vi "Image Dispose.vi"(5 "Archive?":bool, 7 "Dispose?":bool, 8 "error in":errorcluster, 11 "Gluing Procedure in":refnum<class "Gluing Procedure.lvclass">) -> (0 "error out":errorcluster, 3 "Gluing Procedure out":refnum<class "Gluing Procedure.lvclass">)   [LabVIEW 2017, in "Gluing Procedure.lvclass"]
uses:
  Gluing Procedure.lvclass
  Shared Components/Gantry Class/Gantry Class.lvclass
  Shared Components/Config Manager Class/Config Manager Class.lvclass
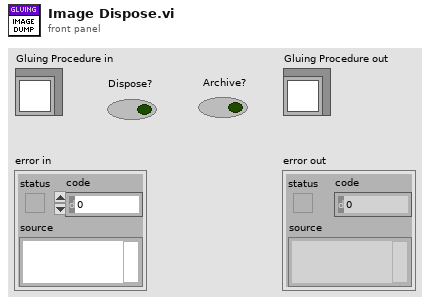
[diagram p1: front panel]
types:
  T1 = typedef "Part Fiducials.ctl" = cluster{"Fiducials":T2[], "Chuck":i32, "Slot":i32}
  T2 = typedef "Fiducial Image.ctl" = cluster{"Fiducial Image":T3, "Selected Fiducial":T5, "fiducial name":string}
  T3 = typedef "Physical Image.ctl" = cluster{"Image Position":refnum<class "Vec3d Class.lvclass">, "Image Reference":T4, "Field of View":cluster{"x(mm)":dbl, "y(mm)":dbl}}
  T4 = typedef "IMAQ Image.ctl" = refnum<image>
  T5 = typedef "Fiducial with Source.ctl" = cluster{"Fiducial Image Coordinate":refnum<class "Vec3d Class.lvclass">, "Fiducial Source":enum16{"Pattern Recognition", "User", "Error", "Default"}}
  T6 = cluster{"HDI Fiducials":T1, "Stamp Fiducials":T1, "Weight Fiducials":T1, "BBM Fiducials":T1}[]
  T7 = cluster{"HDI Fiducials":T1, "Stamp Fiducials":T1, "Weight Fiducials":T1, "BBM Fiducials":T1}
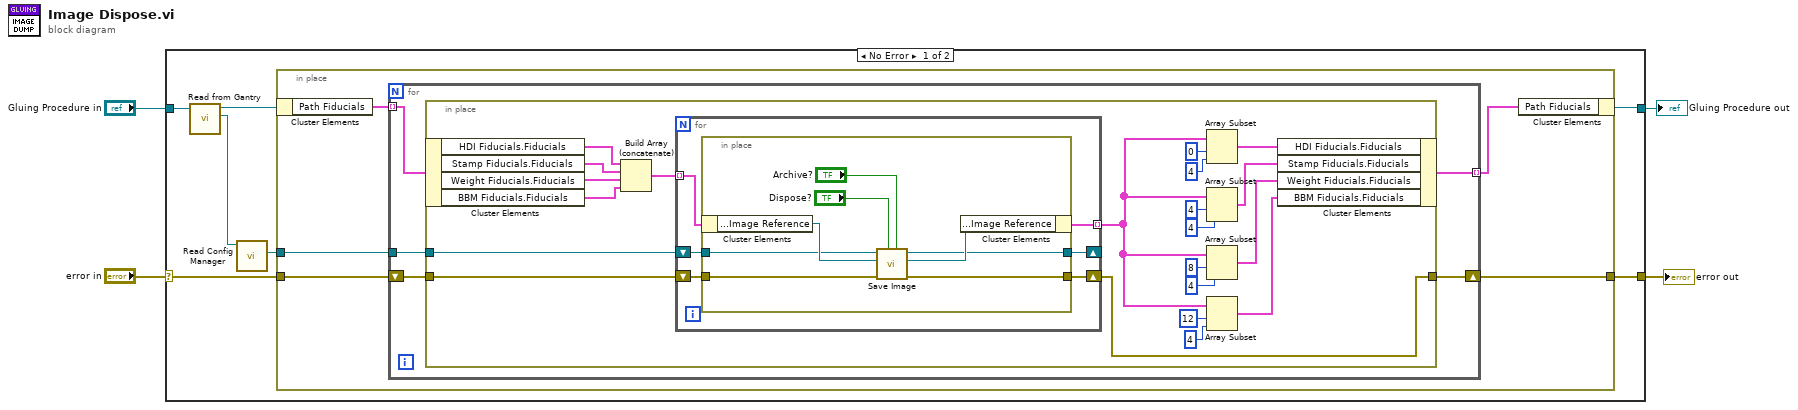
[diagram p0: block diagram]
diagram:
  n1 = case shown="No Error" "error in" {
    selector: "error in" -> [w7 w57]
    tunnel: [w6 w58] -> w2
    tunnel: "Gluing Procedure in" -> [w11 w58]
    tunnel: [w5 w57] -> w1
    frame No Error {
      n2 = call "Read from Gantry.vi"("Gluing Procedure in"=w11) -> ("Gantry"=w10:refnum<class "Gantry Class.lvclass">, "Gluing Procedure out"=w9:refnum<class "Gluing Procedure.lvclass">)  [unwired: 8 in, 1 out]
      n3 = call-dynamic "Read Config Manager.vi"("Gantry in"=w10) -> ("Config Manager"=w8:refnum<class "Config Manager Class.lvclass">)  [unwired: 8 in, 2 out]
      n4 = in-place {
        in-place-border: w8 -> [w15]
        in-place-border: w7 -> [w14]
        in-place-border: [w12] -> w5
        n5 = in-place-cluster #1(w9) -> ("Path Fiducials"=w16:T6)
        n6 = for {
          tunnel: w16 -> [w21] mode=indexing
          tunnel: w15 -> [w20]
          shift-right: [w18] -> w12
          shift-left: w14 -> [w19]
          tunnel: [w17] -> w13 mode=indexing
          n7 = in-place {
            in-place-border: w20 -> [w37]
            in-place-border: w19 -> [w36]
            in-place-border: [w22] -> w18
            n8 = in-place-cluster #2(w21) -> ("HDI Fiducials.Fiducials"=w42:T2[], "Stamp Fiducials.Fiducials"=w41:T2[], "Weight Fiducials.Fiducials"=w40:T2[], "BBM Fiducials.Fiducials"=w39:T2[])
            n9 = Build Array (concatenate)(w42, w41, w40, w39) -> (w38:T2[])
            n10 = for {
              tunnel: w38 -> [w48] mode=indexing
              shift-right: [w44] -> _
              shift-left: w37 -> [w47]
              shift-right: [w45] -> w22
              shift-left: w36 -> [w46]
              tunnel: [w43] -> w35 mode=indexing
              n11 = in-place {
                in-place-border: w47 -> [w52]
                in-place-border: w46 -> [w51]
                in-place-border: [w50] -> w45
                in-place-border: [w49] -> w44
                n12 = in-place-cluster #3(w48) -> ("Fiducial Image.Image Reference"=w56:T4)
                n13 = call "Save Image.vi"("Archive"="Archive?", "Dispose"="Dispose?", "error in"=w51, "Image in"=w56, "Config Manager in"=w52) -> ("error out"=w50:errorcluster, "Image out"=w55:T4, "Config Manager out"=w49:refnum<class "Config Manager Class.lvclass">)  [unwired: 4 in]
                n14 = in-place-cluster #3("Fiducial Image.Image Reference"=w55) -> (w43:T2)
              }
            }
            n15 = Array Subset(array=w35, index=0, length=4) -> (w34:T2[])
            n16 = Array Subset(array=w35, index=4, length=4) -> (w33:T2[])
            n17 = Array Subset(array=w35, index=8, length=4) -> (w32:T2[])
            n18 = Array Subset(array=w35, index=12, length=4) -> (w31:T2[])
            n19 = in-place-cluster #2("HDI Fiducials.Fiducials"=w34, "Stamp Fiducials.Fiducials"=w33, "Weight Fiducials.Fiducials"=w32, "BBM Fiducials.Fiducials"=w31) -> (w17:T7)
          }
        }
        n20 = in-place-cluster #1("Path Fiducials"=w13) -> (w6:refnum<class "Gluing Procedure.lvclass">)
      }
    }
    frame Error {
    }
  }
  "error out" <- w1
  "Gluing Procedure out" <- w2
